vi "Stop Module.vi"(6 "Timeout to Wait for Stop (s) (-1: no timeout)":dbl=-1.0, 8 "error in":errorcluster, 9 "Wait for Module to Stop? (F)":bool, 10 "Origin":string) -> (0 "error out":errorcluster)   [LabVIEW 2018, in "MB switches Module.lvlib"]
doc: "Send the Stop request to the Module's Main.vi.\n\nIf <b>Wait for Module to Stop?</b> is TRUE, this VI will wait until the module main VI stops, and will timeout at the <b>Timeout to Wait for Stop</b> value. This value defaults to \"-1\", which means the VI will not timeout, and will always wait until the module main VI stops before completing execution.\n\nNote: The <b>Timeout to Wait for Stop</b> value is ignored if 'Wait for Module to Stop?' is set to FALSE.\n_____\nBased on DQMH Project Template 6.0.0.91."
uses:
  MB switches Module.lvlib
  Stop Argument--cluster.ctl
  <vilib>/event_ctls.llb/usereventprio.ctl
panel:
  # "Note: The 'Timeout to Wait for Stop' value is ignored if 'Wait for Module to Stop?' is set to FALSE."
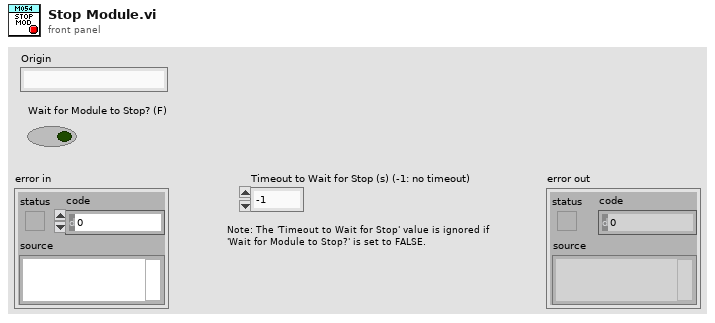
[diagram p1: front panel]
types:
  T1 = typedef "MB switches Module.lvlib/Stop Argument--cluster.ctl" = cluster{"Origin":string, "Exit via Stop Module Req?":bool, "Wait for Module to stop?":bool}
  T2 = typedef "usereventprio.ctl" = enum32{"high priority", "normal priority"}
  T3 = typedef "MB switches Module.lvlib/Request Events--cluster.ctl" = cluster{"Stop Module":refnum<user-event>, "Do Something Else and Wait for Reply":refnum<user-event>, "Show Panel":refnum<user-event>, "Hide Panel":refnum<user-event>, "Get Module Execution Status":refnum<user-event>, "Show Diagram":refnum<user-event>, "inst.Counter":refnum<user-event>, "inst.Open":refnum<user-event>, "inst.Close":refnum<user-event>, "inst.Optos":refnum<user-event>, "mux10-1_chan0":refnum<user-event>, "mux6-1_chan0":refnum<user-event>, "DMM I 0.5_10":refnum<user-event>, "mux10-1_chan1":refnum<user-event>, "mux10-1_chan2":refnum<user-event>, "mux10-1_chan3":refnum<user-event>, "mux10-1_chan4":refnum<user-event>, "mux10-1_chan5":refnum<user-event>, "mux10-1_chan6":refnum<user-event>, "mux10-1_chan7":refnum<user-event>, "mux10-1_chan8":refnum<user-event>, "mux10-1_chan9":refnum<user-event>, "mux10-1_chan10":refnum<user-event>, "mux6-1_chan1_1":refnum<user-event>, "mux6-1_chan1_2":refnum<user-event>, "mux6-1_chan2_1":refnum<user-event>, "mux6-1_chan2_2":refnum<user-event>}
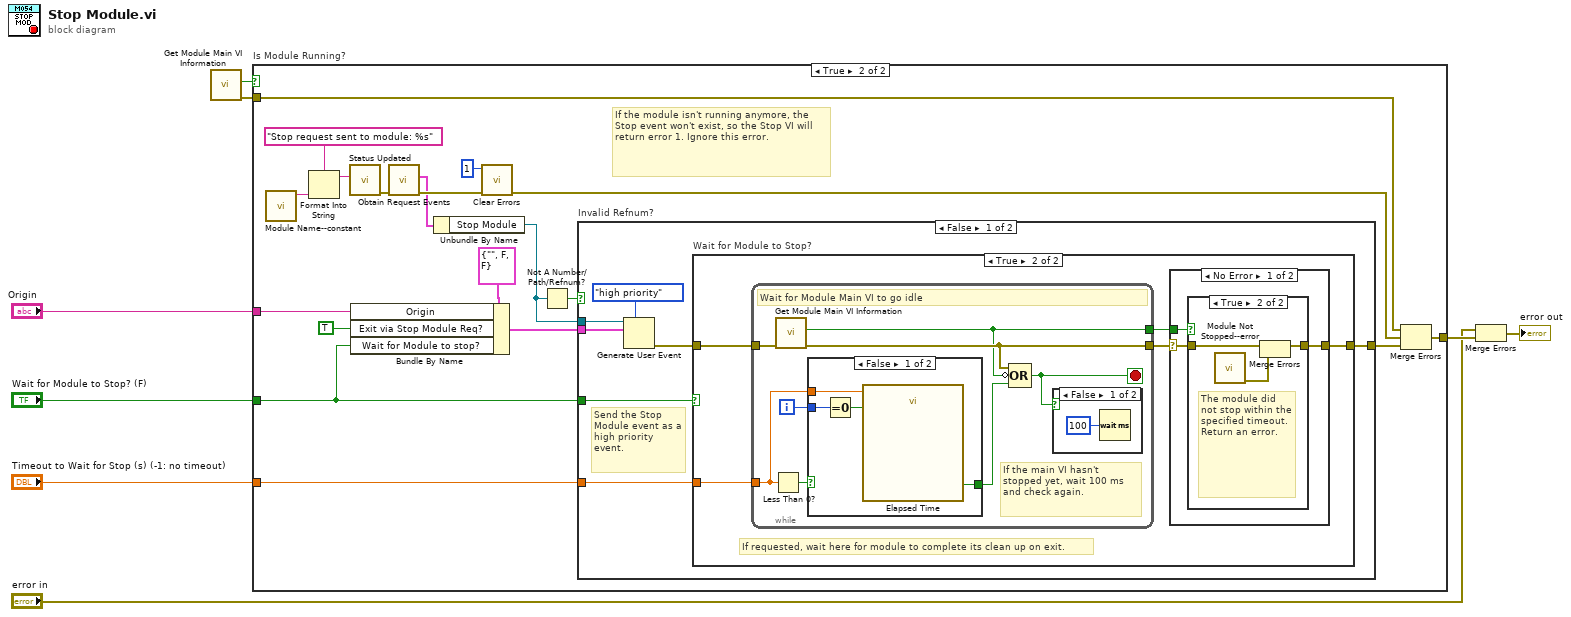
[diagram p0: block diagram]
diagram:
  n1 = call "Get Module Main VI Information.vi"() -> ("error out"=w5:errorcluster, "Is Module Running?"=w4:bool)  [unwired: 8 in, 2 out]
  n2 = case "Is Module Running?" shown="True" w4 {
    tunnel: [w9 w27] -> w8
    tunnel: "Origin" -> [_ w26]
    tunnel: w5 -> [w9 w15]
    tunnel: "Wait for Module to Stop? (F)" -> [_ w11]
    tunnel: "Timeout to Wait for Stop (s) (-1: no timeout)" -> [_ w10]
    frame False {
      # "The module is not running, there is no need to run the Stop Module code."
    }
    frame True {
      # "If the module isn't running anymore, the Stop event won't exist, so the Stop VI will return error 1. Ignore this error."
      n3 = call "Module Name--constant.vi"() -> ("Module Name"=w22:string)  [unwired: 11 in]
      n4 = Format Into String(format string="Stop request sent to module: %s", w22) -> (resulting string=w23:string)  [unwired: 2 in, 1 out]
      n5 = call "Status Updated.vi"("Status"=w23) -> ("error out"=w14:errorcluster)  [unwired: 10 in]
      n6 = Bundle By Name(cluster=T1 {"Origin"="", "Exit via Stop Module Req?"=FALSE, "Wait for Module to stop?"=FALSE} ("event data"), "Origin"=w26, "Exit via Stop Module Req?"=TRUE, "Wait for Module to stop?"=w11) -> (w18:T1)
      n7 = call "Obtain Request Events.vi"("error in (no error)"=w14) -> ("error out"=w28:errorcluster, "Switches Module Request Events"=w25:T3)  [unwired: 9 in]
      n8 = Unbundle By Name(w25) -> ("Stop Module"=w19:refnum<user-event>)
      n9 = call <vilib>:"Clear Errors.vi"("error in (no error)"=w28, "specific error code to clear (0: all)"=1) -> ("error out"=w13:errorcluster)  [unwired: 4 in, 1 out]
      n10 = Not A Number/Path/Refnum?(number/path/refnum=w19) -> (NaN/Path/Refnum?=w20:bool)
      n11 = case "Invalid Refnum?" shown="False" w20 {
        tunnel: [w30 _] -> w17
        tunnel: w19 -> [w35 _]
        tunnel: w18 -> [w33 _]
        tunnel: w11 -> [w31 _]
        tunnel: w10 -> [w29 _]
        frame False {
          # "Send the Stop Module event as a high priority event."
          n12 = Generate User Event(priority (normal)=usereventprio."high priority", user event=w35, event data cluster=w33) -> (error out=w32:errorcluster)  [unwired: 1 in, 1 out]
          n13 = case "Wait for Module to Stop?" shown="True" w31 {
            tunnel: w32 -> [w36 w40]
            tunnel: [w36 w38] -> w30
            tunnel: w29 -> [_ w41]
            frame False {
            }
            frame True {
              # "If requested, wait here for module to complete its clean up on exit."
              n14 = while {
                tunnel: w41 -> [w52]
                tunnel: w40 -> [w56]
                tunnel: [w55] -> w39
                tunnel: [w54] -> w37
                i -> [w57]
                stop <- w50 stop-if-true
                # "If the main VI hasn't stopped yet, wait 100 ms and check again."
                # "Wait for Module Main VI to go idle"
                n15 = Less Than 0?(x=w52) -> (x < 0?=w51:bool)
                n16 = call "Get Module Main VI Information.vi"("error in (no error)"=w56) -> ("error out"=w55:errorcluster, "Is Module Running?"=w54:bool)  [unwired: 7 in, 2 out]
                n17 = case shown="False" w51 {
                  tunnel: w52 -> [w59 _]
                  tunnel: w57 -> [w61 _]
                  tunnel: [w60 _] -> w53
                  frame False {
                    n18 = Equal To 0?(x=w61) -> (x = 0?=w62:bool)
                    n19 = call "Elapsed Time"("Time Target (s)"=w59, "Reset"=w62) -> ("Time has Elapsed"=w60:bool)  [unwired: 10 in, 7 out]
                  }
                  frame True {
                    # "User specified a timeout of -1, so don't keep track of the elapsed time since this loop started."
                  }
                }
                n20 = Compound Arithmetic op=OR(w55, invert w54, w53) -> (w50:bool)
                n21 = case shown="False" w50 {
                  frame False {
                    n22 = Wait (ms)(milliseconds to wait=u32 100) -> ()  [unwired: 1 out]
                  }
                  frame True {
                  }
                }
              }
              n23 = case shown="No Error" w39 {
                selector: w39 -> [w43 w49]
                tunnel: [w42 w49] -> w38
                tunnel: w37 -> [w44 _]
                frame No Error {
                  n24 = case shown="True" w44 {
                    tunnel: w43 -> [w45 w48]
                    tunnel: [w45 w47] -> w42
                    frame False {
                      # "The module stopped, and no error occurred."
                    }
                    frame True {
                      # "The module did not stop within the specified timeout. Return an error."
                      n25 = call "Module Not Stopped--error.vi"() -> ("error out"=w46:errorcluster)  [unwired: 11 in]
                      n26 = Merge Errors(w48, w46) -> (w47:errorcluster)
                    }
                  }
                }
                frame Error {
                  # "An error occurred while waiting for the module to stop. Return that error."
                }
              }
            }
          }
        }
        frame True {
          # "Module is exiting. No need to send the standard \"not running\" error that is sent in other request VIs."
        }
      }
      n27 = Merge Errors(w15, w13, w17) -> (w27:errorcluster)
    }
  }
  n28 = Merge Errors("error in", w8) -> (→"error out":errorcluster)
